vi "GRC Route.vi"() -> ()   [LabVIEW 2020]
uses:
  Source/Protobuf RAW/int32/int32.lvclass/int32.ctl
  Source/Protobuf RAW/int32/Write Value.vi
  Source/Protobuf RAW/int32/int32.lvclass
  E:/Labview/LV 2020/Libs/LV Protobuf Raw/Source/Protobuf RAW/Tag/Basic Type.lvclass
  Source/Protobuf RAW/Message/New Raw Message.vi
  <vilib>/NI/Advanced HTTP Client/POST (Buffer).vi
  Source/Protobuf RAW/Message/Raw Message.lvclass
  Source/Protobuf RAW.lvlib
  E:/Labview/LV 2020/Libs/LV Protobuf Raw/Source/Protobuf RAW/Proto Value/Proto Type.lvclass
  E:/Labview/LV 2020/Libs/LV Protobuf Raw/Source/Protobuf RAW/Type Serializer/Type Serializer.lvclass
  E:/Labview/LV 2020/Libs/LV Protobuf Raw/Source/Protobuf RAW/String Representable/String Representable.lvclass
  E:/Labview/LV 2020/Libs/LV Protobuf Raw/Source/Protobuf RAW/Wire Type Group/Wire Type Group.lvclass
  E:/Labview/LV 2020/Libs/LV Protobuf Raw/Source/Protobuf RAW/Scalar Encoder/Scalar Type.lvclass
  E:/Labview/LV 2020/Libs/LV Protobuf Raw/Source/Protobuf RAW/VarINT Encoder/VarINT.lvclass
  E:/Labview/LV 2020/Libs/LV Protobuf Raw/Source/Protobuf RAW/int32/int32.lvclass
  <vilib>/NI/Advanced HTTP Client/Session.lvclass
panel:
  out "body":string
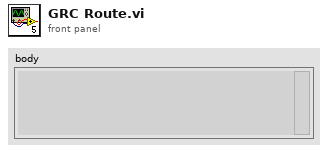
[diagram p1: front panel]
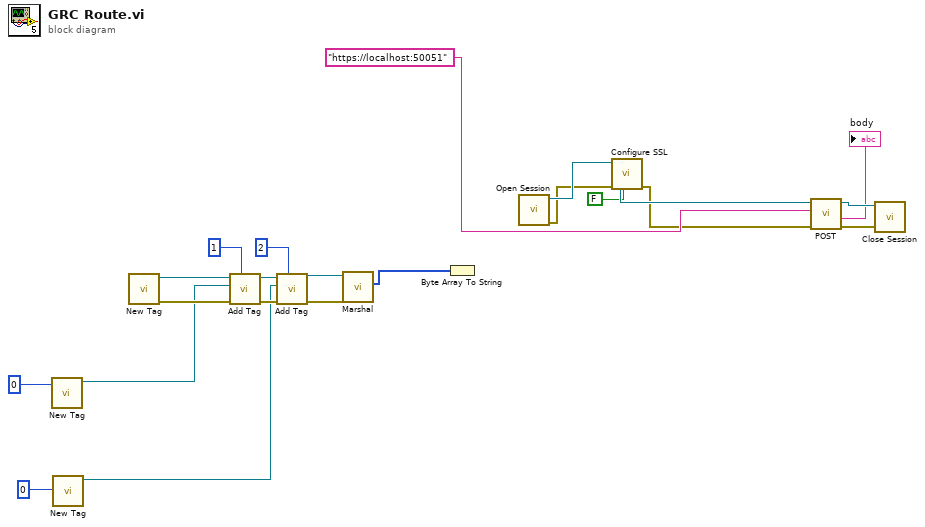
[diagram p0: block diagram]
diagram:
  n1 = call-poly "New Tag.vi"("Value"=0 ("Long")) -> ("int32 out"=w18:refnum<class "int32.lvclass">)  [unwired: 9 in, 1 out]
  n2 = call-poly "New Tag.vi"("Value"=0 ("Lat")) -> ("int32 out"=w17:refnum<class "int32.lvclass">)  [unwired: 9 in, 1 out]
  n3 = call-poly "New Tag.vi"() -> ("error out"=w21:errorcluster, "Raw Message out"=w22:refnum<class "Raw Message.lvclass">)  [unwired: 10 in]
  n4 = call-dynamic "Add Tag.vi"("ID"=u32 1, "error in (no error)"=w21, "Tag Value"=w18, "Message in"=w22) -> ("error out"=w19:errorcluster, "Message out"=w20:refnum<class "Raw Message.lvclass">)  [unwired: 6 in]
  n5 = call-dynamic "Add Tag.vi"("ID"=u32 2, "error in (no error)"=w19, "Tag Value"=w17, "Message in"=w20) -> ("error out"=w13:errorcluster, "Message out"=w14:refnum<class "Raw Message.lvclass">)  [unwired: 6 in]
  n6 = call-dynamic "Marshal.vi"("error in (no error)"=w13, "Message in"=w14) -> ("Buffer"=w10:u8[])  [unwired: 7 in, 2 out]
  n7 = Byte Array To String(unsigned byte array=w10) -> ()  [unwired: 1 out]
  n8 = call <vilib>:"Open Session.vi"() -> ("error out"=w3:errorcluster, "session"=w6:refnum<class "Session.lvclass">)  [unwired: 10 in]
  n9 = call <vilib>:"Configure SSL.vi"("verify server"=FALSE, "error in"=w3, "session in"=w6) -> ("error out"=w2:errorcluster, "session out"=w5:refnum<class "Session.lvclass">)  [unwired: 7 in]
  n10 = call-poly <vilib>:"POST.vi"("error in"=w2, "url"="https://localhost:50051", "session in"=w5) -> ("error out"=w1:errorcluster, "body"=→"body":string, "session out"=w9:refnum<class "Session.lvclass">)  [unwired: 4 in, 2 out]
  n11 = call <vilib>:"Close Session.vi"("error in"=w1, "session"=w9) -> ()  [unwired: 9 in, 1 out]
